vi "Check for Win.vi"(8 "error in (no error)":errorcluster, 11 "Reversi in":refnum<class "Reversi.lvclass">) -> (0 "error out":errorcluster, 2 "Any Moves Left?":bool, 3 "Reversi out":refnum<class "Reversi.lvclass">)   [LabVIEW 2020, in "Reversi.lvlib" / "Reversi.lvclass"]
uses:
  Reversi.lvclass
  Reversi.lvclass/Reversi.ctl
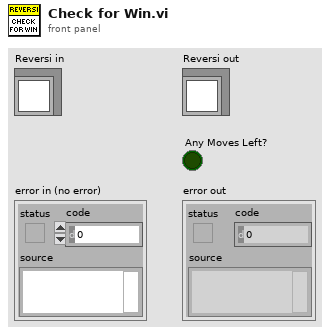
[diagram p1: front panel]
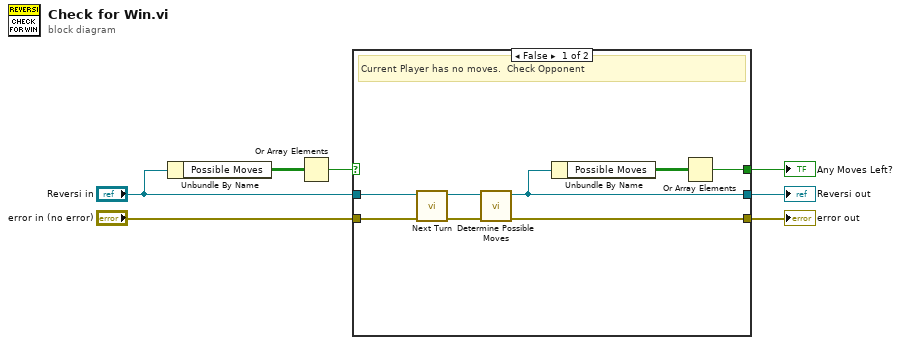
[diagram p0: block diagram]
diagram:
  n1 = Unbundle By Name("Reversi in") -> ("Possible Moves"=w7:bool[][])
  n2 = Or Array Elements(Boolean array=w7) -> (logical OR=w6:bool)
  n3 = case shown="False" w6 {
    selector: w6 -> [_ w18]
    tunnel: "Reversi in" -> [w15 w17]
    tunnel: "error in (no error)" -> [w12 w16]
    tunnel: [w11 w18] -> w1
    tunnel: [w9 w16] -> w3
    tunnel: [w8 w17] -> w2
    frame False {
      # "Current Player has no moves.  Check Opponent"
      n4 = call "Next Turn.vi"("error in (no error)"=w12, "Reversi in"=w15) -> ("error out"=w10:errorcluster, "Reversi out"=w14:refnum<class "Reversi.lvclass">)  [unwired: 8 in]
      n5 = call "Determine Possible Moves.vi"("error in (no error)"=w10, "Reversi in"=w14) -> ("error out"=w9:errorcluster, "Reversi out"=w8:refnum<class "Reversi.lvclass">)  [unwired: 8 in]
      n6 = Unbundle By Name(w8) -> ("Possible Moves"=w13:bool[][])
      n7 = Or Array Elements(Boolean array=w13) -> (logical OR=w11:bool)
    }
    frame True {
      # "Current Player has moves."
    }
  }
  "error out" <- w3
  "Reversi out" <- w2
  "Any Moves Left?" <- w1
